vi "GetAttributeViBoolean_SS-DMod_ListSeq_RF.vi"(8 "error in (no error)":errorcluster {"code" format="%.0x"}, 9 "AttributeID":u32(ring)=1150917 items=["SS_DIGITALMODULATION_ARB_ENABLED"=1150917, "SS_DIGITALMODULATION_ARB_EXTERNAL_TRIGGER_DELAY_ENABLED"=1150886, "SS_DIGITALMODULATION_ARB_IQADJUSTMENT_ENABLED"=1150918, "SS_DIGITALMODULATION_ARB_SEQUENCE_SYNC_ENABLED"=1150907, "SS_LISTSEQUENCER_ENABLED"=1150903, "SS_RFGENERATOR_MODULATION_AM_ENABLED"=1150927, "SS_RFGENERATOR_MODULATION_ENABLED"=1150940, "SS_RFGENERATOR_MODULATION_FM_ENABLED"=1150930, "SS_RFGENERATOR_MODULATION_PM_ENABLED"=1150932, "SS_RFGENERATOR_OUTPUT_ENABLED"=1150942, "SS_RFGENERATOR_REFERENCE_FREQUENCY_ENABLED"=1150913, "SS_RFGENERATOR_REFERENCE_POWER_ENABLED"=1150915], 10 "RepCapIdentifier":string, 11 "instrument handle":refnum<k15>) -> (0 "error out":errorcluster {"code" format="%.0x"}, 2 "AttributeValue":bool, 3 "instrument handle out":refnum<k15>)   [LabVIEW 2009, in "Keysight XSAn.lvlib"]
doc: "Gets a Boolean attribute from the instrument driver.\nThe following Attributes are supported:\n\nSS_DIGITALMODULATION_ARB_ENABLED\nSS_DIGITALMODULATION_ARB_EXTERNAL_TRIGGER_DELAY_ENABLED\nSS_DIGITALMODULATION_ARB_IQADJUSTMENT_ENABLED\nSS_DIGITALMODULATION_ARB_SEQUENCE_SYNC_ENABLED\nSS_LISTSEQUENCER_ENABLED\nSS_RFGENERATOR_MODULATION_AM_ENABLED\nSS_RFGENERATOR_MODULATION_ENABLED\nSS_RFGENERATOR_MODULATION_FM_ENABLED\nSS_RFGENERATOR_MODULATION_PM_ENABLED\nSS_RFGENERATOR_OUTPUT_ENABLED\nSS_RFGENERATOR_REFERENCE_FREQUENCY_ENABLED\nSS_RFGENERATOR_REFERENCE_POWER_ENABLED"
uses:
  <instrlib>/Keysight XSAn/Keysight XSAn.lvlib
  AgXSAn.dll
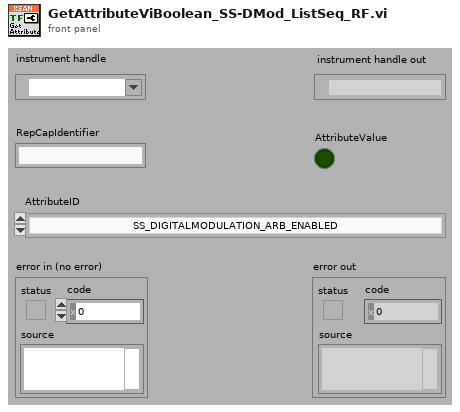
[diagram p1: front panel]
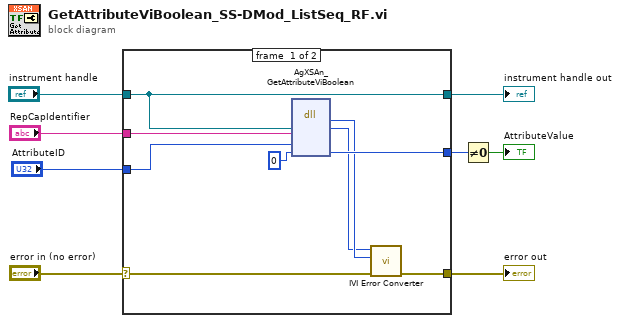
[diagram p0: block diagram]
diagram:
  n1 = case shown="No Error" "error in (no error)" {
    selector: "error in (no error)" -> [w17 w19]
    tunnel: [w16 w19] -> w8
    tunnel: "instrument handle" -> [w11 w18]
    tunnel: "RepCapIdentifier" -> [w15 _]
    tunnel: "AttributeID" -> [w14 _]
    tunnel: [w12 _] -> w3
    tunnel: [w11 w18] -> w2
    frame #0 {
      n2 = dll-call lib="AgXSAn**.dll" fn="AgXSAn_GetAttributeViBoolean"("Vi"=w11, "RepCapIdentifier"=w15, "AttributeID"=w14, "AttributeValue"=i16 0) -> ("return type"=w10:i32, "Vi"=w9:u32, "AttributeValue"=w12:i16)  [unwired: 5 in, 2 out]
      n3 = call <instrlib>:"IVI Error Converter.vi"("error in (no error)"=w17, "IVI error code (0)"=w10, "instrument handle"=w9) -> ("error out"=w16:errorcluster)  [unwired: 7 in, 1 out]
    }
    frame #1 {
    }
  }
  "error out" <- w8
  "instrument handle out" <- w2
  n4 = Not Equal To 0?(x=w3) -> (x != 0?=→"AttributeValue":bool)
